vi "2.3.vi"() -> ()   [LabVIEW 2020]
panel:
  in  "stop":bool
  out "temperatura alcanzada":bool
  out "termometro":dbl(slide) scale=25.0..90.0
  out "tanque":dbl(slide) scale=0.0..100.0
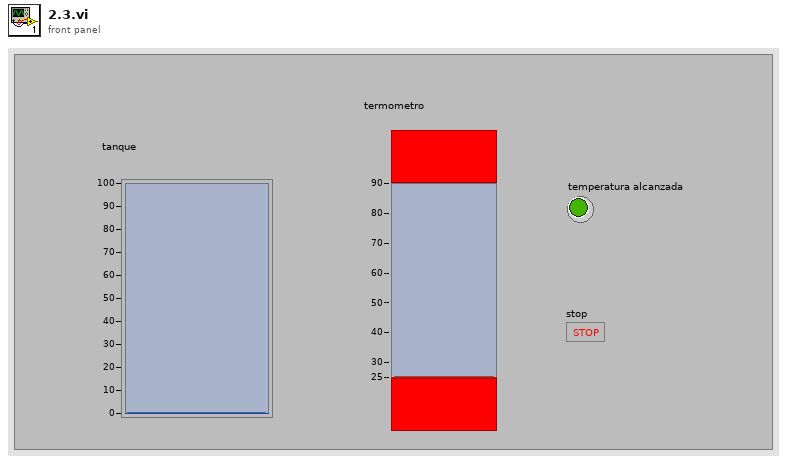
[diagram p1: front panel]
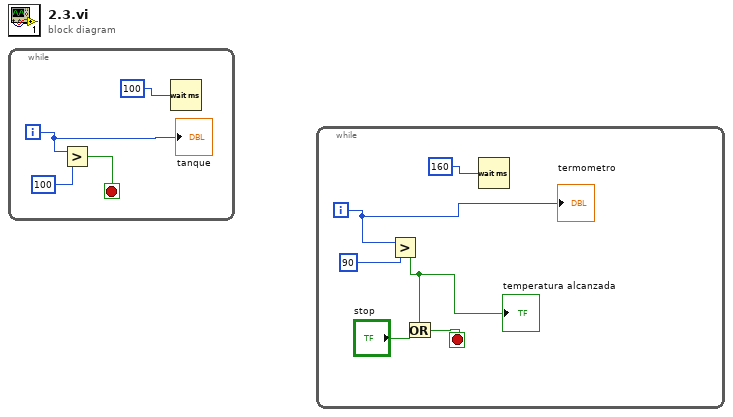
[diagram p0: block diagram]
diagram:
  n1 = while {
    i -> [w3]
    stop <- w2 stop-if-true
    n2 = Greater?(x=w3, y=100) -> (0:w2:bool)
    n3 = Wait (ms)(milliseconds to wait=100) -> ()  [unwired: 1 out]
    "tanque" <- w3
  }
  n4 = while {
    i -> [w8]
    stop <- w7 stop-if-true
    n5 = Greater?(x=w8, y=90) -> (0:w5:bool)
    "temperatura alcanzada" <- w5
    n6 = Or(x=w5, y="stop") -> (x .or. y?=w7:bool)
    n7 = Wait (ms)(milliseconds to wait=160) -> ()  [unwired: 1 out]
    "termometro" <- w8
  }
